vi "Write Last Frame Time.vi"(8 "error in (no error)":errorcluster, 10 "Last Frame Time":timestamp, 11 "PhysicsSystem in":refnum<class "PhysicsSystem.lvclass">) -> (0 "error out":errorcluster, 3 "PhysicsSystem out":refnum<class "PhysicsSystem.lvclass">)   [LabVIEW 2022 SP3, in "PhysicsSystem.lvclass"]
uses:
  PhysicsSystem.lvclass
  PhysicsSystem.lvclass/PhysicsSystem.ctl
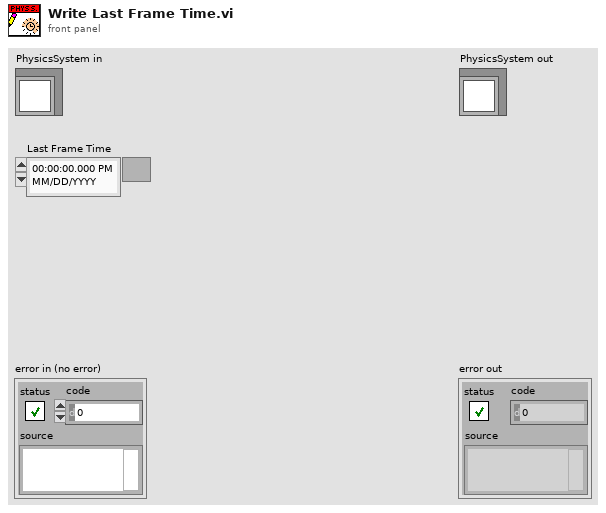
[diagram p1: front panel]
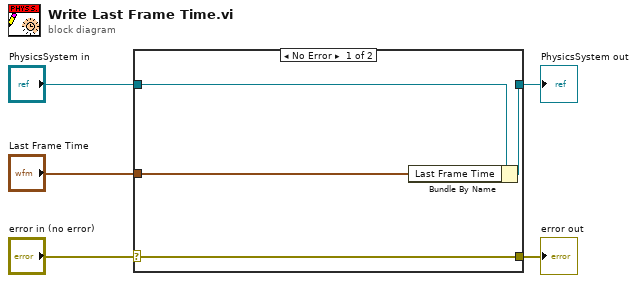
[diagram p0: block diagram]
diagram:
  n1 = case shown="No Error" "error in (no error)" {
    selector: "error in (no error)" -> [w9 w10]
    tunnel: [w9 w10] -> w4
    tunnel: [w7 w11] -> w2
    tunnel: "PhysicsSystem in" -> [w8 w11]
    tunnel: "Last Frame Time" -> [w6 _]
    frame No Error {
      n2 = Bundle By Name(cluster=w8, "Last Frame Time"=w6) -> (w7:refnum<class "PhysicsSystem.lvclass">)
    }
    frame Error {
    }
  }
  "error out" <- w4
  "PhysicsSystem out" <- w2
